vi "test Cluster Set and Get.vi"(8 "error in (no error)":errorcluster, 11 "TestCase in":refnum<class "AIM ARINC 664 Scripting.lvclass">) -> (0 "error out":errorcluster, 3 "TestCase out":refnum<class "AIM ARINC 664 Scripting.lvclass">)   [LabVIEW 2020, in "AIM ARINC 664 Scripting.lvclass"]
uses:
  AIM ARINC 664 Scripting.lvclass
  C:/Program Files (x86)/National Instruments/LabVIEW 2020/vi.lib/addons/_JKI Toolkits/VI Tester/TestCase.llb/TestCase.lvclass
  <vilib>/addons/_JKI Toolkits/VI Tester/TestCase.llb/TestCase.lvclass
  Scripting/AIM ARINC 664 Scripting.lvlib
  <vilib>/addons/database/_DB Variant To Data/Database Variant To Data.xnode
panel:
  out "data":T1
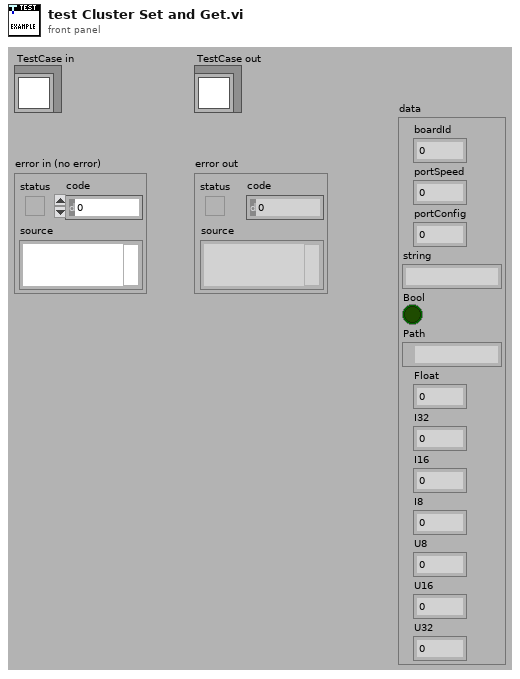
[diagram p1: front panel]
types:
  T1 = cluster{"boardId":u32, "portSpeed":u32, "portConfig":u32, "string":string, "Bool":bool, "Path":path, "Float":dbl, "I32":i32, "I16":i16, "I8":i8, "U8":u8, "U16":u16, "U32":u32}
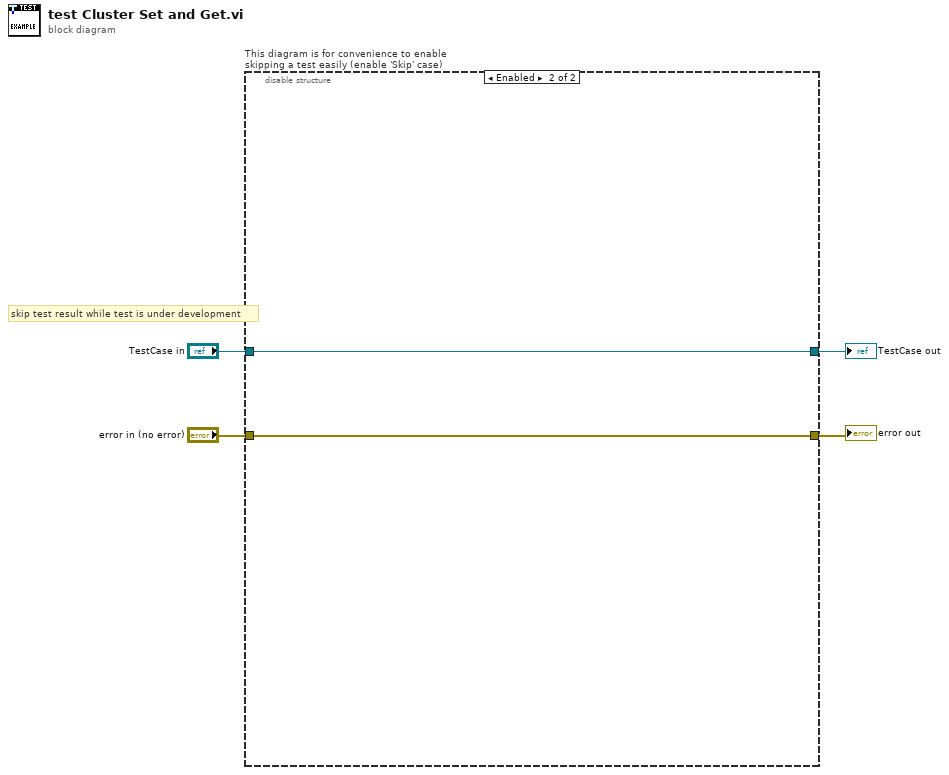
[diagram p0: block diagram]
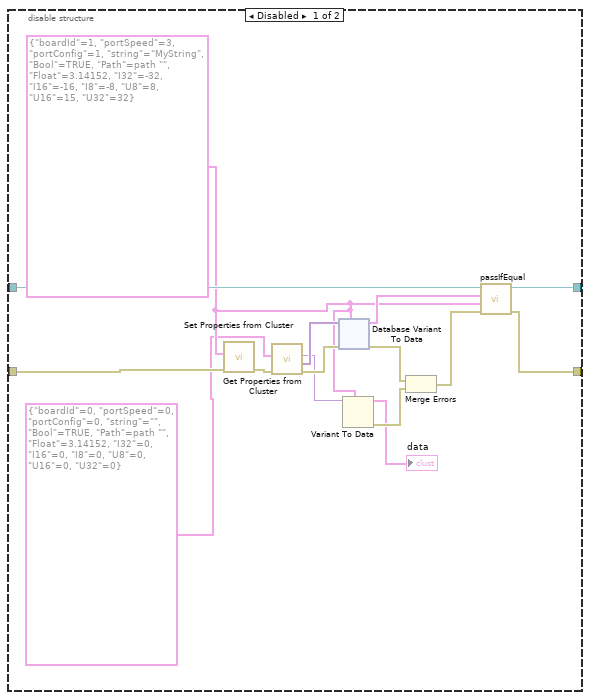
[diagram p2: hidden frame]
diagram:
  n1 = disable-structure "This diagram is for convenience to enable skipping a test easily (enable 'Skip' case)" shown="Enabled" {
    disable-tunnel: "TestCase in" -> [w17 w430]
    disable-tunnel: [w18 w428] -> w1
    disable-tunnel: [w19 w429] -> w3
    disable-tunnel: "error in (no error)" -> [w16 w427]
    frame Disabled {
      w10 = T1 {"boardId"=1, "portSpeed"=3, "portConfig"=1, "string"="MyString", "Bool"=TRUE, "Path"=path "", "Float"=3.14152, "I32"=-32, "I16"=-16, "I8"=-8, "U8"=8, "U16"=15, "U32"=32} ("boardSetup")
      n2 = call "Set Properties from Cluster.vi"("error in"=w16, "Variant Cluster"=w10) -> ("error out"=w15:errorcluster)  [unwired: 8 in, 1 out]
      n3 = call "Get Properties from Cluster.vi"("error in"=w15, "Variant Cluster"=T1 {"boardId"=0, "portSpeed"=0, "portConfig"=0, "string"="", "Bool"=TRUE, "Path"=path "", "Float"=3.14152, "I32"=0, "I16"=0, "I8"=0, "U8"=0, "U16"=0, "U32"=0} ("boardSetup")) -> ("error out"=w14:errorcluster, "Array"=w12:variant[], "data"=w11:variant)  [unwired: 6 in, 1 out]
      n4 = xnode "Database Variant To Data"("database variant"=w12, "error in (no error)"=w14, "type"=w10) -> ("data"=w13:T1, "error out"=w8:errorcluster)
      n5 = Variant To Data(type=w10, Variant=w11) -> (data=→"data":T1, error out=w6:errorcluster)  [unwired: 1 in]
      n6 = Merge Errors(w8, w6) -> (w7:errorcluster)
      n7 = call-dynamic "passIfEqual.vi"("error in (no error)"=w7, "y"=w10, "x"=w13, "TestCase in"=w17) -> ("error out"=w19:errorcluster, "TestCase out"=w18:refnum<class "AIM ARINC 664 Scripting.lvclass">)  [unwired: 6 in]
    }
    frame Enabled {
      # "skip test result while test is under development"
      n8 = call <vilib>:"skip.vi"("error in (no error)"=w427, "TestCase in"=w430) -> ("error out"=w429:errorcluster, "TestCase out"=w428:refnum<class "AIM ARINC 664 Scripting.lvclass">)  [unwired: 8 in]
    }
  }
  "error out" <- w3
  "TestCase out" <- w1
